vi "GetChannels.vi"(8 "error in (no error)":errorcluster, 11 "FgenPluginsBase in":refnum<class "FgenPluginsBase.lvclass">) -> (0 "error out":errorcluster, 2 "Channels":cluster{"Count":u16, "Channel":T1[]}, 3 "FgenPluginsBase out":refnum<class "FgenPluginsBase.lvclass">)   [LabVIEW 2018, in "FgenPlugins.lvlib" / "FgenPluginsBase.lvclass"]
uses:
  FgenPluginsBase.lvclass
  TypeDefs/Channel.ctl
  FgenPluginsBase.lvclass/FgenPluginsBase.ctl
  Accessors/Read Channels.vi
  FgenPlugins.lvlib
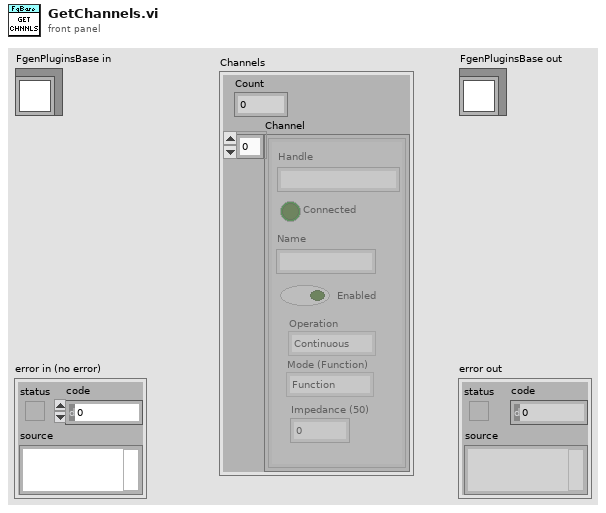
[diagram p1: front panel]
types:
  T1 = typedef "FgenPlugins.lvlib/Channel.ctl" = cluster{"Name":string, "Enabled":bool, "Operation":enum16{"Continuous", "Burst"}, "Impedance (50)":dbl, "Handle":string, "Connected":bool, "Mode (Function)":enum16{"Function", "Arbitrary", "Sequence"}}
  T2 = typedef "Channel.ctl" = cluster{"Name":string, "Enabled":bool, "Operation":enum16{"Continuous", "Burst"}, "Impedance (50)":dbl, "Handle":string, "Connected":bool, "Mode (Function)":enum16{"Function", "Arbitrary", "Sequence"}}
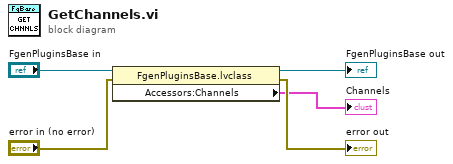
[diagram p0: block diagram]
diagram:
  n1 = property class="FgenPluginsBase.lvclass"(reference="FgenPluginsBase in", error in="error in (no error)") -> (reference out=→"FgenPluginsBase out":refnum<class "FgenPluginsBase.lvclass">, error out=→"error out":errorcluster, "Accessors:Channels"=→"Channels":cluster{"Count":u16, "Channel":T2[]})
